vi "运行剖面至指定位置.vi"(8 "error in (no error)":errorcluster, 10 "停止":bool, 11 "位置设置值":dbl) -> (0 "error out":errorcluster, 3 "定位完成":bool)   [LabVIEW 2016, in "elevator.lvlib"]
uses:
  elevator.lvlib
  main/main.lvlib
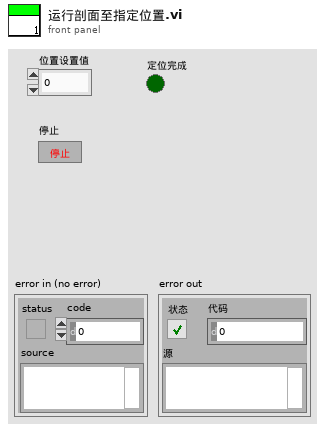
[diagram p1: front panel]
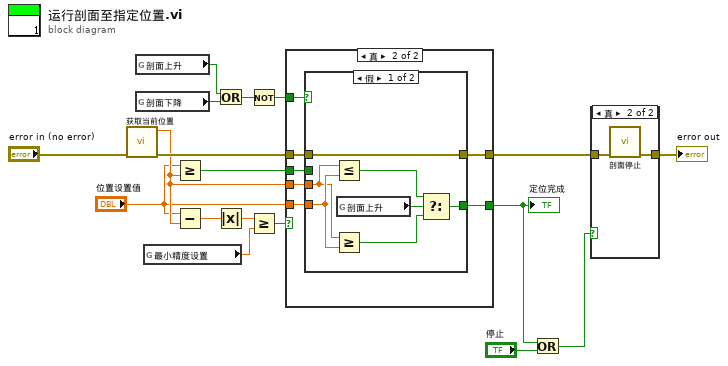
[diagram p0: block diagram]
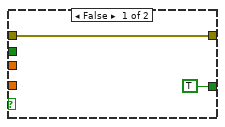
[diagram p3: hidden frame]
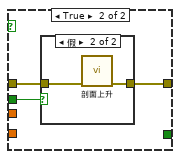
[diagram p4: hidden frame]
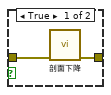
[diagram p5: hidden frame]
diagram:
  n1 = call "获取当前位置.vi"("error in (no error)"="error in (no error)") -> ("error out"=w17:errorcluster, "编码器工程量"=w7:dbl)  [unwired: 8 in, 1 out]
  n2 = global read "全局非断电保持变量.vi" "剖面上升"() -> (w4:bool)
  n3 = global read "全局非断电保持变量.vi" "剖面下降"() -> (w5:bool)
  n4 = global read "全局断电保存变量.vi" "最小精度设置"() -> (w1:dbl)
  n5 = Greater Or Equal?(x="位置设置值", y=w7) -> (x >= y?=w18:bool)
  n6 = Subtract(x="位置设置值", y=w7) -> (x-y=w16:dbl)
  n7 = Or(x=w4, y=w5) -> (x .or. y?=w3:bool)
  n8 = Absolute Value(x=w16) -> (abs(x)=w15:dbl)
  n9 = Not(x=w3) -> (.not. x?=w2:bool)
  n10 = Greater Or Equal?(x=w15, y=w1) -> (x >= y?=w14:bool)
  n11 = case shown="真" w14 {
    tunnel: w18 -> [_ w27]
    tunnel: w17 -> [w19 w26]
    tunnel: [TRUE w22] -> w12
    tunnel: [w19 w25] -> w10
    tunnel: w7 -> [_ w24]
    tunnel: "位置设置值" -> [_ w23]
    tunnel: w2 -> [_ w21]
    frame False {
    }
    frame True {
      n12 = case shown="假" w21 {
        tunnel: w27 -> [_ w37]
        tunnel: w26 -> [w31 w36]
        tunnel: [w31 w35] -> w25
        tunnel: w24 -> [w28 _]
        tunnel: w23 -> [w29 _]
        tunnel: [w30 _] -> w22
        frame False {
          n13 = Less Or Equal?(x=w28, y=w29) -> (x <= y?=w33:bool)
          n14 = Greater Or Equal?(x=w28, y=w29) -> (x >= y?=w32:bool)
          n15 = global read "全局非断电保持变量.vi" "剖面上升"() -> (w34:bool)
          n16 = Select(t=w33, s=w34, f=w32) -> (s? t:f=w30:bool)
        }
        frame True {
          n17 = case shown="假" w37 {
            tunnel: w36 -> [w38 w40]
            tunnel: [w39 w41] -> w35
            frame True {
              n18 = call "剖面下降.vi"("error in (no error)"=w38) -> ("error out"=w39:errorcluster)  [unwired: 10 in]
            }
            frame False {
              n19 = call "剖面上升.vi"("error in (no error)"=w40) -> ("error out"=w41:errorcluster)  [unwired: 10 in]
            }
          }
        }
      }
    }
  }
  "定位完成" <- w12
  n20 = Or(x=w12, y="停止") -> (x .or. y?=w11:bool)
  n21 = case shown="真" w11 {
    tunnel: w10 -> [w42 w44]
    tunnel: [w42 w43] -> w8
    frame False {
    }
    frame True {
      n22 = call "剖面停止.vi"("error in (no error)"=w44) -> ("error out"=w43:errorcluster)  [unwired: 10 in]
    }
  }
  "error out" <- w8
